vi "SIM_FreqShiftOutput.vi"(11 "zin (m)":dbl) -> (3 "Current Out (pA)":dbl)   [LabVIEW 2019]
uses:
  <vilib>/ptbypt/NI_PtbyPt.lvlib
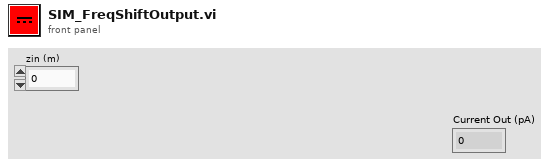
[diagram p1: front panel]
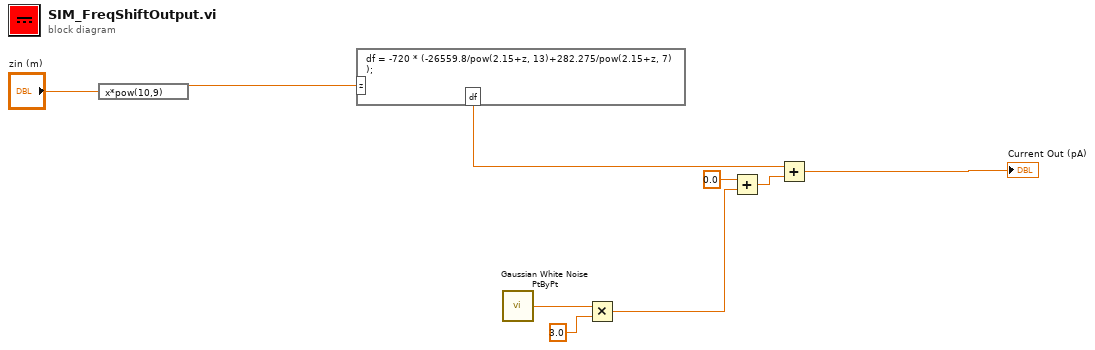
[diagram p0: block diagram]
diagram:
  n1 = expression code="x*pow(10,9)"("zin (m)") -> (w2:dbl)
  n2 = formula code="df = -720 * (-26559.8/pow(2.15+z, 13)+282.275/pow(2.15+z, 7) );"("z"=w2) -> ("df"=w4:dbl)
  n3 = call <vilib>:"Gaussian White Noise PtByPt.vi"() -> ("Gaussian white noise"=w9:dbl)  [unwired: 3 in]
  n4 = Multiply(x=w9, y=3.0) -> (x*y=w6:dbl)
  n5 = Add(x=0.0, y=w6) -> (x+y=w7:dbl)
  n6 = Add(x=w4, y=w7) -> (x+y=→"Current Out (pA)":dbl)
